vi "Check.vi"(8 "error in (no error)":errorcluster) -> (0 "error out":errorcluster, 2 "Passed":bool)   [LabVIEW 2017, in "WebServiceImporter.lvlib" / "Main Panel.lvlib" / "Select Methods.lvlib"]
uses:
  <vilib>/Platform/WebService/Main Panel/Pages/Select Methods/Select Methods.lvlib
  <vilib>/Platform/WebService/Main Panel/Events/Events.lvlib
  <vilib>/Platform/WebService/Main Panel/Pages/Select Methods/Events/Events.lvlib
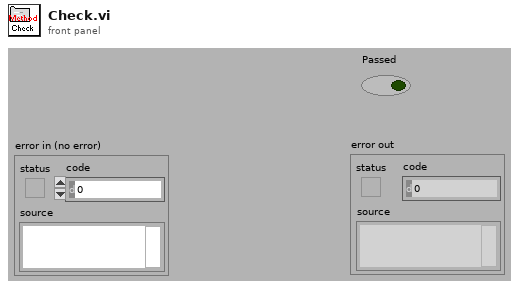
[diagram p1: front panel]
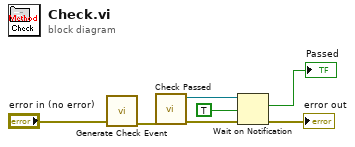
[diagram p0: block diagram]
diagram:
  n1 = call <vilib>:"Generate Check Event.vi"("error in (no error)"="error in (no error)") -> ("error out"=w2:errorcluster)  [unwired: 10 in]
  n2 = call <vilib>:"Check Passed.vi"("error in (no error)"=w2) -> ("error out"=w3:errorcluster, "notifier  (out)"=w5:refnum<notifier>)  [unwired: 9 in]
  n3 = Wait on Notification(notifier=w5, ignore previous (F)=TRUE, error in (no error)=w3) -> (notification=→"Passed":bool, error out=→"error out":errorcluster)  [unwired: 1 in, 2 out]
